vi "Autonomous Independent_04042012.vi"() -> ()   [LabVIEW 2011]
doc: "This VI is called when autonomous begins, and will automatically be terminated when autonomous ends. You can carry out timed or sensor driven robot movement independently without needing to return to the caller."
uses:
  <vilib>/Rock Robotics/WPI/Joystick/WPI_JoystickButtonState.ctl
  Robot Global Data.vi
  <vilib>/addons/control/pid/pid.llb/PID (DBL).vi
  <vilib>/Rock Robotics/WPI/RobotDrive/WPI_RobotDriveArcadeDrive_Standard(NoSaturation).vi
  <vilib>/addons/control/pid/NI_PID_pid.lvlib
panel:
  in  "Forward_Time_Cntrl_2_s2_p0":i32(slide) scale=0.0..100.0
  in  "Turn_Time_Cntrl_s2_p0":i32(slide) scale=0.0..100.0
  in  "Backward_Time_Cntrl_s2_p0":i32(slide) scale=0.0..100.0
  in  "Shooting_Time_Cntrl_s2_p0":u32(slide) scale=0.0..100.0
  in  "Shooting_Time_Cntrl_s1_p1":u32(slide) scale=0.0..100.0
  in  "Forward_Time_Cntrl_1_s1_p1":i32(slide) scale=0.0..100.0
  in  "Backward_Time_Cntrl_s1_p1":i32(slide) scale=0.0..100.0
  in  "Turn_Time_Cntrl_s1_p1":i32(slide) scale=0.0..100.0
  in  "Forward_Time_Cntrl_2_s1_p1":i32(slide) scale=0.0..100.0
  in  "Forward_Time_Cntrl_2_s1_p0":i32(slide)=15 scale=0.0..100.0
  in  "Turn_Time_Cntrl_s1_p0":i32(slide)=25 scale=0.0..100.0
  in  "Backward_Time_Cntrl_s1_p0":i32(slide)=81 scale=0.0..100.0
  in  "Forward_Time_Cntrl_1_s1_p0":i32(slide)=55 scale=0.0..100.0
  in  "Shooting_Time_Cntrl_s1_p0":u32(slide)=42 scale=0.0..100.0
  in  "Shooter_Speed_Cntrl":dbl(slide)=0.65 scale=-1.0..1.0
  in  "ARM_FWD_LIMIT":dbl(slide)=0.53 scale=1.0..-1.0
  in  "ARM_REV_LIMIT":dbl(slide)=-0.14110429447852763 scale=1.0..-1.0
  in  "ARM_HOME":dbl(slide)=0.53 scale=1.0..-1.0
  in  "Feeder_Arm_Speed":dbl
  out "JS1_BTNS":T1
  out "JS1_AXES":T2
  in  "Kinect_Arm_Conrol":dbl
  out "Kinect_Drive_Reduce":dbl=0.5
  out "KINECT_BTNS":T1
  out "LEFT_ARM_AXES":T2
  out "RIGHT_ARM_AXES":T2
  in  "Ball_Sucker_Speed":dbl(slide)=0.6 scale=-1.0..1.0
  in  "Feed_Speed_Cntrl":dbl(slide)=0.9 scale=-1.0..1.0
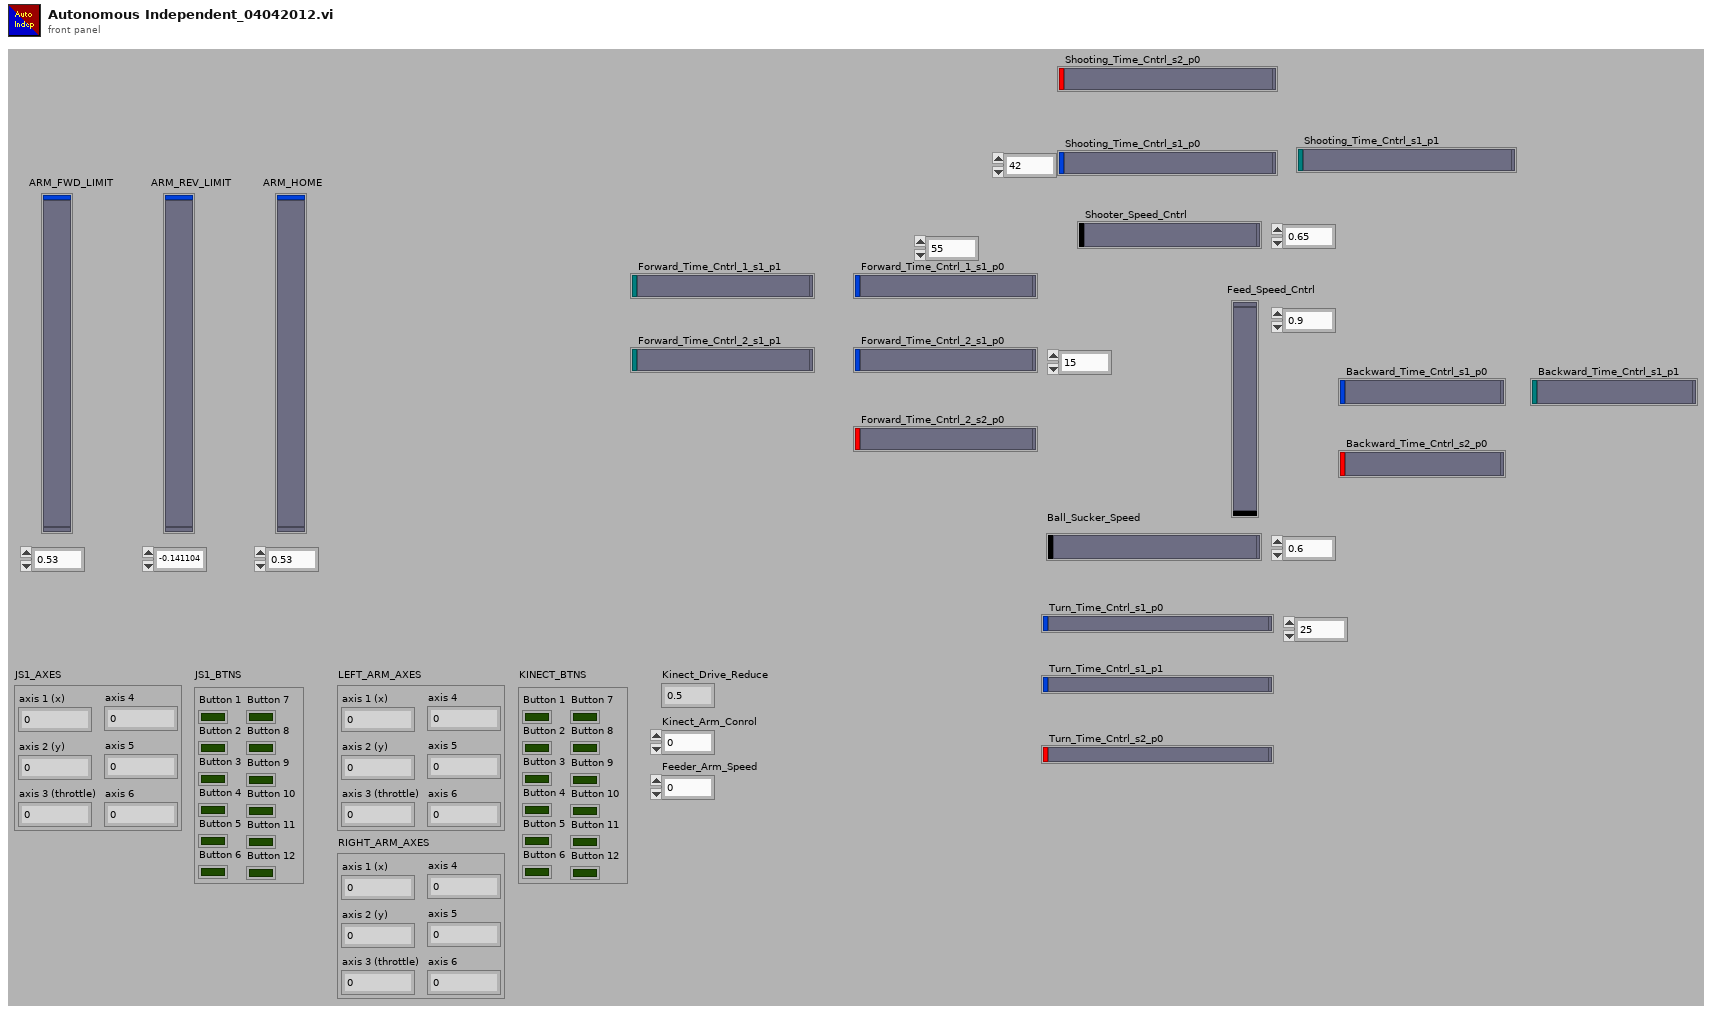
[diagram p1: front panel]
types:
  T1 = typedef "WPI_JoystickButtonState.ctl" = cluster{"Button 1":bool, "Button 2":bool, "Button 3":bool, "Button 4":bool, "Button 5":bool, "Button 6":bool, "Button 7":bool, "Button 8":bool, "Button 9":bool, "Button 10":bool, "Button 11":bool, "Button 12":bool}
  T2 = cluster{"axis 1 (x)":dbl, "axis 2 (y)":dbl, "axis 3 (throttle)":dbl, "axis 4":dbl, "axis 5":dbl, "axis 6":dbl}
  T3 = cluster{"proportional gain (Kc)":dbl, "integral time (Ti, min)":dbl, "derivative time (Td, min)":dbl}
  T4 = typedef "WPI_RobotDriveDevRef.ctl" = cluster{"DevStatus":errorcluster, "Motors[]":T5[], "Square Inputs":bool, "Max Output":dbl, "Isochronous":bool}
  T5 = typedef "WPI_MotorControlDeviceRef.ctl" = cluster{"DeviceStatus":errorcluster, "Type":enum16{"PWM", "CAN"}, "PWM":cluster{"Digital Module":T6, "PWM Channel":T7, "DeadBand":T8}, "CAN":cluster{"Device Number":u8, "Control Mode":T9, "Semaphore":T10, "Max Vout":dbl}, "Invert":bool, "TransformRef":T11, "InvTransformRef":T11}
  T6 = typedef "FPGA_TypedefDigitalModule.ctl" = enum16{"Digital Module 1", "Digital Module 2"}
  T7 = typedef "FPGA_DIOPWMChannel.ctl" = enum8{"PWM 1", "PWM 2", "PWM 3", "PWM 4", "PWM 5", "PWM 6", "PWM 7", "PWM 8", "PWM 9", "PWM 10", "Invalid"}
  T8 = typedef "WPI_PWMDeadband.ctl" = cluster{"Name":string, "maxPositivePwm":i32, "minPositivePwm":i32, "centerPwm":i32, "maxNegativePwm":i32, "minNegativePwm":i32, "angularRange":u16}
  T9 = typedef "WPI_CANJaguar_ControlMode.ctl" = enum8{"Percent VBus", "Current", "Speed", "Position", "Voltage"}
  T10 = typedef "Semaphore RefNum" = refnum<k1>
  T11 = typedef "WPI_PWMTransform_ConPane.ctl" = refnum<vi>
  T12 = typedef "WPI_JoystickDevRef.ctl" = cluster{"Device":T13}
  T13 = typedef "WPI_JoystickDeviceEnum.ctl" = enum16{"USB 1", "USB 2", "USB 3", "USB 4", "Kinect 1", "Kinect 2"}
  T14 = typedef "WPI_AnalogChannelDevRef.ctl" = cluster{"DevStatus":errorcluster, "Analog Module":T15, "Analog Channel":T16}
  T15 = typedef "FPGA_TypedefAnalogModule.ctl" = enum16{"Analog Module 1", "Analog Module 2"}
  T16 = typedef "FPGA_AIChannel.ctl" = enum8{"AI 1", "AI 2", "AI 3", "AI 4", "AI 5", "AI 6", "AI 7", "AI 8", "Invalid"}
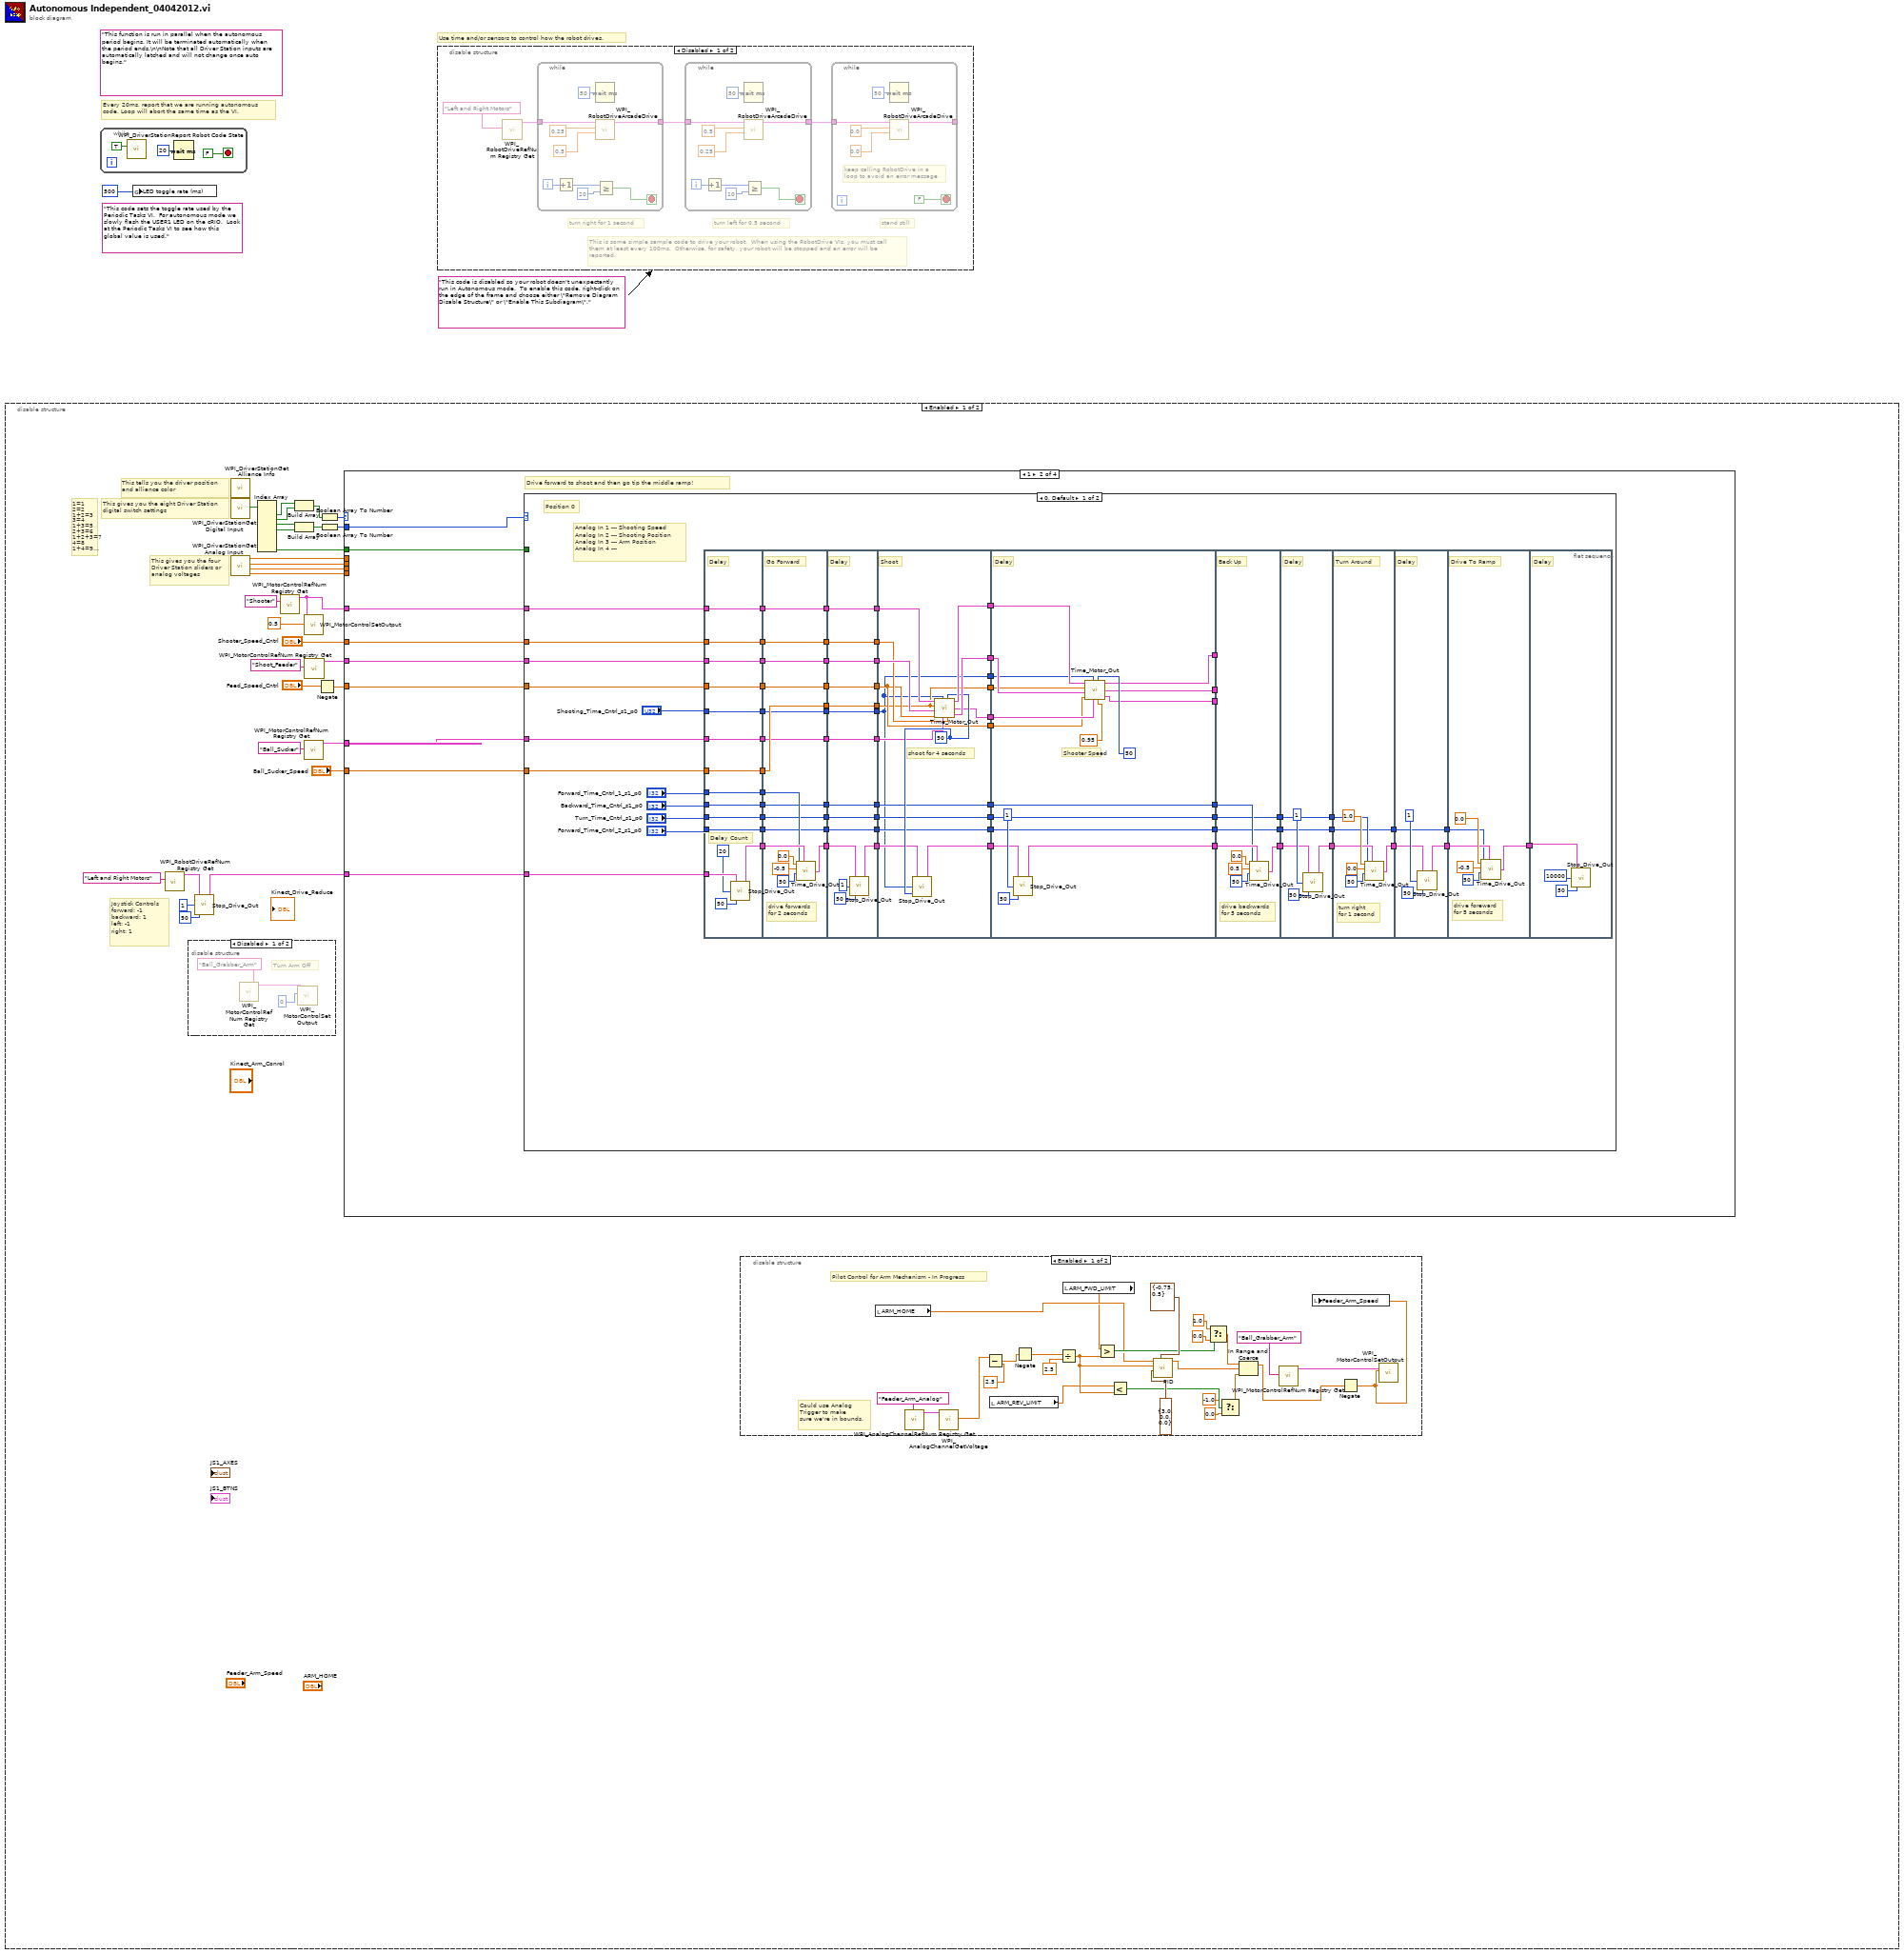
[diagram p0: block diagram]
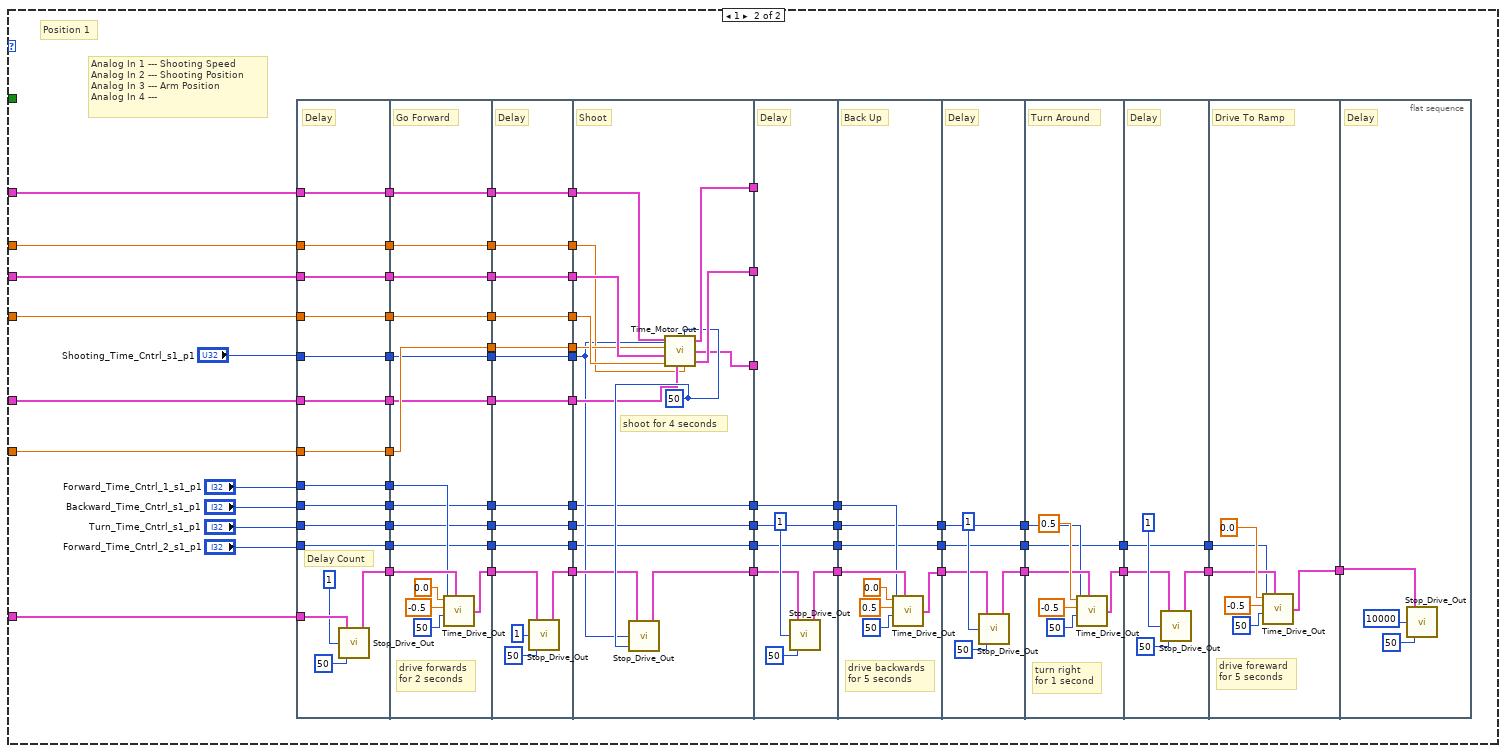
[diagram p5: hidden frame]
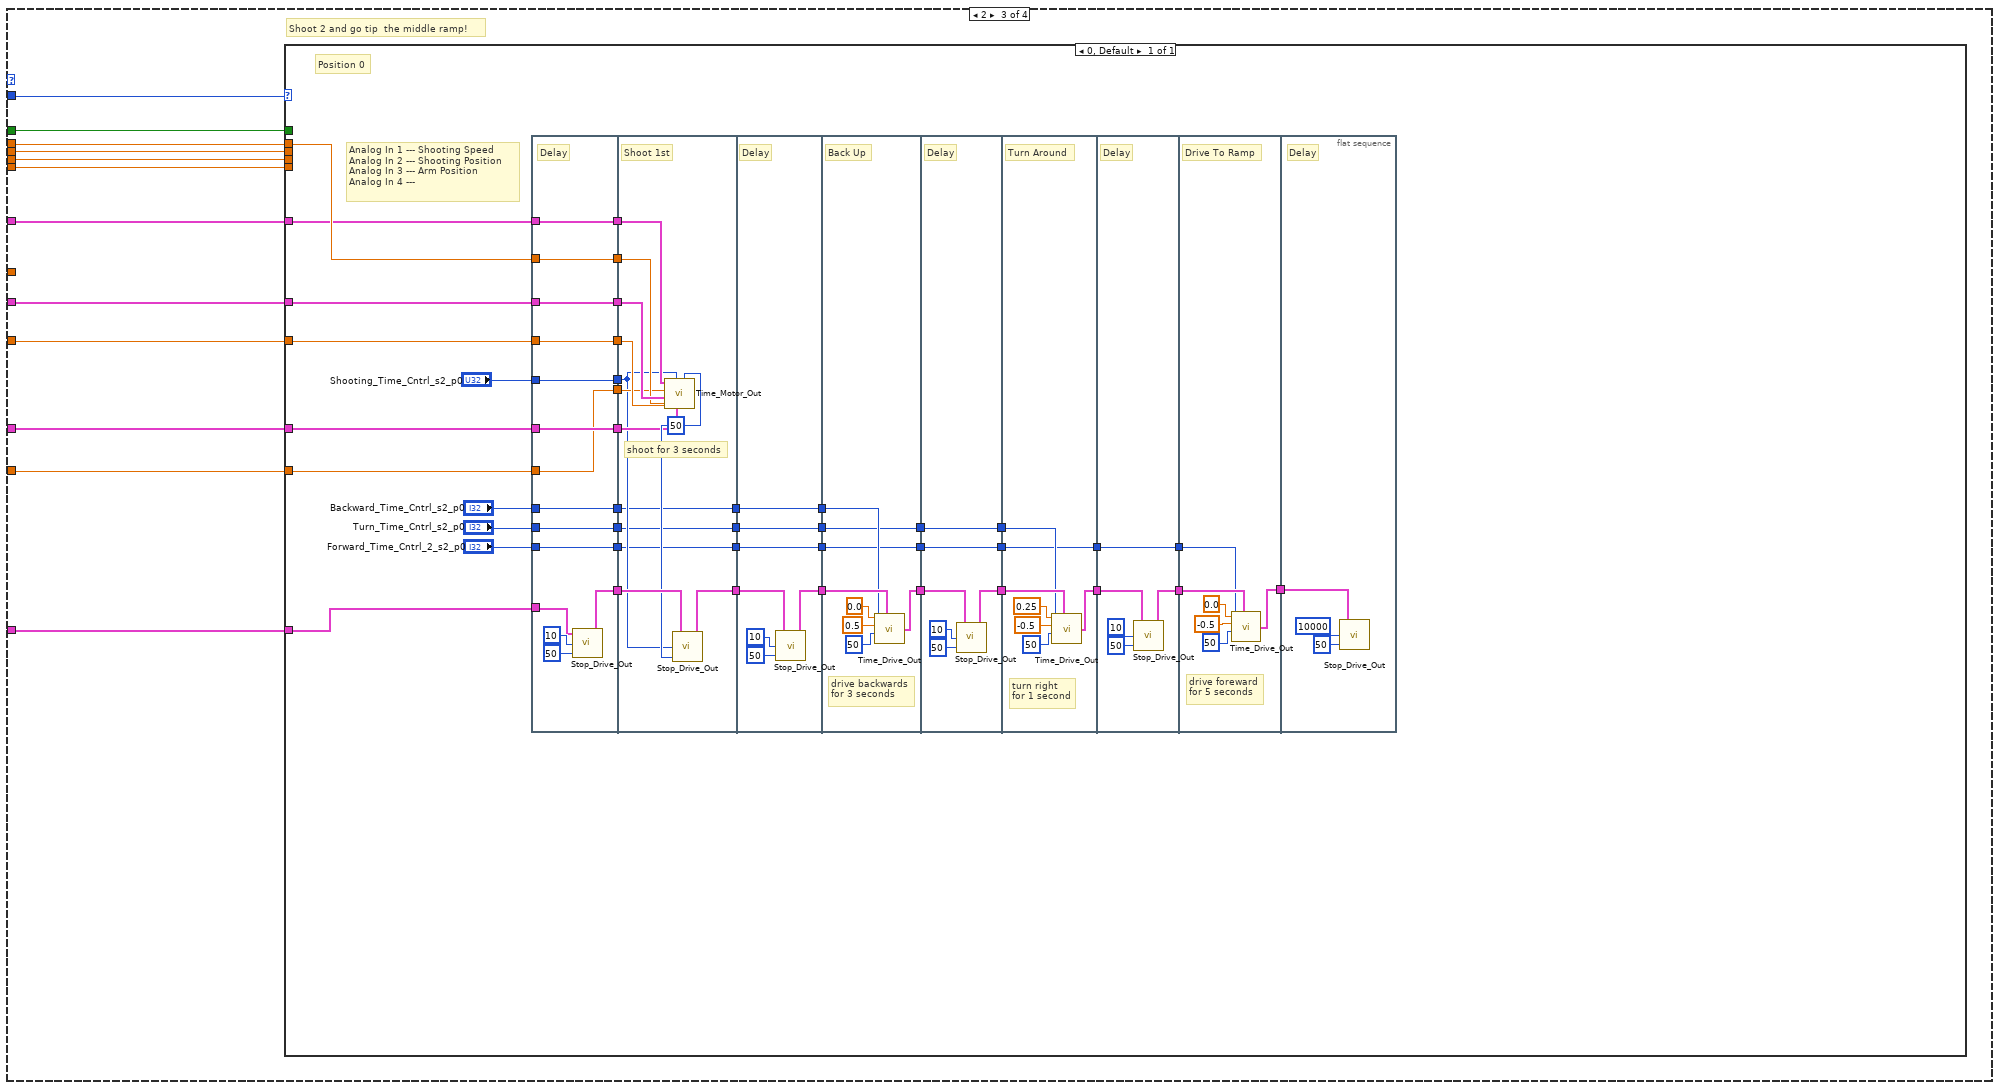
[diagram p6: hidden frame]
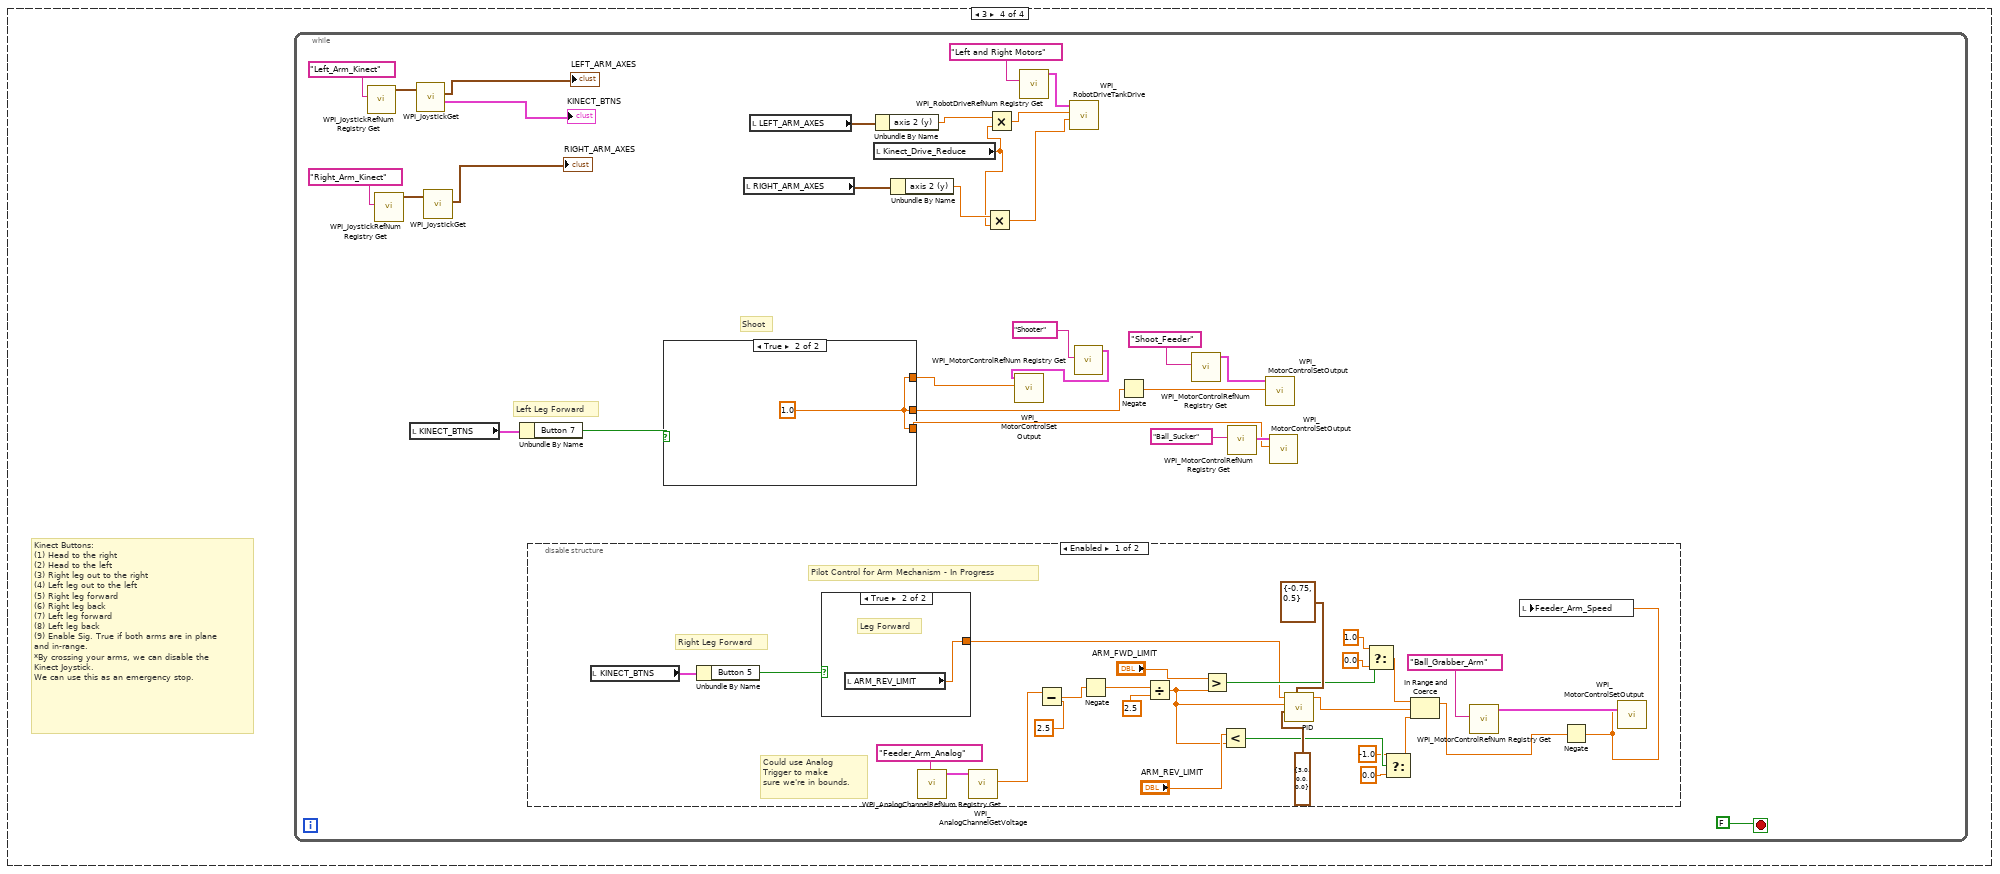
[diagram p7: hidden frame]
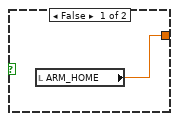
[diagram p8: hidden frame]
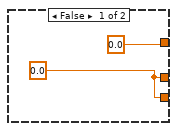
[diagram p10: hidden frame]
diagram:
  (unwired) "This code sets the toggle rate used by the Periodic Tasks VI.  For autonomous mode we slowly flash the USER1 LED on the cRIO.  Look at the Periodic Tasks VI to see how this global value is used."
  (unwired) "This code is disabled so your robot doesn't unexpectantly run in Autonomous mode.  To enable this code, right-click on the edge of the frame and choose either \"Remove Diagram Disable Structure\" or \"Enable This Subdiagram\"."
  (unwired) "This function is run in parallel when the autonomous period begins. It will be terminated automatically when the period ends.\n\nNote that all Driver Station inputs are automatically latched and will not change once auto begins."
  # "Every 20ms, report that we are running autonomous\ncode. Loop will abort the same time as the VI."
  # "Use time and/or sensors to control how the robot drives."
  n1 = disable-structure shown="Enabled" {
    frame Enabled {
      # "Joystick Controls\nforward: -1\nbackward: 1\nleft: -1\nright: 1"
      # "1=1\n2=2\n1+2=3\n3=4\n1+3=5\n2+3=6\n1+2+3=7\n4=8\n1+4=9\n2+4=10\n1+2+4=11\n3+4=12\n1+3+4=13\n2+3+4=14\n1+2+3+4=15"
      # "This tells you the driver position\nand alliance color"
      # "This gives you the eight Driver Station\ndigital switch settings"
      # "This gives you the four\nDriver Station sliders or\nanalog voltages"
      n2 = call <vilib>:"WPI_RobotDriveRefNum Registry Get.vi"("refnum name"="Left and Right Motors") -> ("RobotDriveDevRef"=w13:T4)  [unwired: 1 in, 9 out]
      n3 = disable-structure shown="Disabled" {
        frame Disabled {
          # "Turn Arm Off"
          n4 = call <vilib>:"WPI_MotorControlRefNum Registry Get.vi"("refnum name"="Ball_Grabber_Arm") -> ("MotorControlDevRef"=w60:T5)  [unwired: 1 in, 9 out]
          n5 = call <vilib>:"WPI_MotorControlSetOutput.vi"("Output"=0, "MotorControlDevRef"=w60) -> ()  [unwired: 3 in, 7 out]
        }
        frame Enabled {
        }
      }
      n6 = call "Stop_Drive_Out.vi"("Step_Duration_ms"=50, "Num_Steps"=u32 1 ("milliseconds to wait"), "Drive_In"=w13) -> ("Drive_Out"=w12:T4)
      n7 = call <vilib>:"WPI_DriverStationGet Alliance Info.vi"() -> ()  [unwired: 12 out]
      n8 = call <vilib>:"WPI_DriverStationGet Digital Input.vi"() -> ("Driver Station Digital Input (1-8)"=w31:bool[])  [unwired: 11 out]
      n9 = call <vilib>:"WPI_DriverStationGet Analog Input.vi"() -> ("Analog 4 (V)"=w28:dbl, "Analog 3 (V)"=w29:dbl, "Analog 2 (V)"=w16:dbl, "Analog 1 (V)"=w17:dbl)  [unwired: 8 out]
      n10 = Index Array(array=w31) -> (element #1=w20:bool, element #2=w19:bool, element #3=w22:bool, element #4=w21:bool, element #8=w27:bool)  [unwired: 8 in, 3 out]
      n11 = call <vilib>:"WPI_MotorControlRefNum Registry Get.vi"("refnum name"="Shooter") -> ("MotorControlDevRef"=w3:T5)  [unwired: 9 in, 1 out]
      n12 = Build Array(w20, w19) -> (w18:bool[])
      n13 = Build Array(w22, w21) -> (w30:bool[])
      n14 = call <vilib>:"WPI_MotorControlSetOutput.vi"("Output"=0.5, "MotorControlDevRef"=w3) -> ()  [unwired: 8 in, 2 out]
      n15 = call <vilib>:"WPI_MotorControlRefNum Registry Get.vi"("refnum name"="Ball_Sucker") -> ("MotorControlDevRef"=w6:T5)  [unwired: 9 in, 1 out]
      n16 = call <vilib>:"WPI_MotorControlRefNum Registry Get.vi"("refnum name"="Shoot_Feeder") -> ("MotorControlDevRef"=w24:T5)  [unwired: 9 in, 1 out]
      n17 = Negate(x="Feed_Speed_Cntrl") -> (-x=w8:dbl)
      n18 = Boolean Array To Number(Boolean array=w18) -> (number=w11:u32)
      n19 = Boolean Array To Number(Boolean array=w30) -> (number=w10:u32)
      n20 = case shown="1" w11 {
        tunnel: w17 -> [_ _ w439 _]
        tunnel: w16 -> [_ _ w438 _]
        tunnel: w29 -> [_ _ w437 _]
        tunnel: w28 -> [_ _ w436 _]
        tunnel: w27 -> [_ w69 w440 _]
        tunnel: w8 -> [_ w68 w435 _]
        tunnel: w3 -> [_ w67 w434 _]
        tunnel: w24 -> [_ w66 w433 _]
        tunnel: w12 -> [_ w65 w432 _]
        tunnel: w10 -> [_ w64 w431 _]
        tunnel: w6 -> [_ w63 w429 _]
        tunnel: "Ball_Sucker_Speed" -> [_ w62 w430 _]
        tunnel: "Shooter_Speed_Cntrl" -> [_ w61 _ _]
        frame 0, Default {
          # "Stop Motors"
        }
        frame 1 {
          # "Drive forward to shoot and then go tip the middle ramp!"
          n21 = case shown="0, Default" w64 {
            tunnel: w69 -> [_ _]
            tunnel: w68 -> [w143 w325]
            tunnel: w67 -> [w142 w324]
            tunnel: w66 -> [w141 w323]
            tunnel: w65 -> [w140 w322]
            tunnel: w63 -> [w139 w321]
            tunnel: w62 -> [w138 w320]
            tunnel: w61 -> [w106 w288]
            frame 0, Default {
              # "Analog In 1 --- Shooting Speed\nAnalog In 2 --- Shooting Position\nAnalog In 3 --- Arm Position\nAnalog In 4 ---"
              # "Position 0"
              n22 = flat-sequence {
                tunnel: [w153] -> w137
                tunnel: [w158] -> w136
                tunnel: [w157] -> w135
                tunnel: [w156] -> w134
                tunnel: [w155] -> w133
                tunnel: w142 -> [w156]
                tunnel: w141 -> [w157]
                tunnel: w106 -> [w155]
                tunnel: w143 -> [w158]
                tunnel: w140 -> [w152]
                tunnel: [w151] -> w132
                tunnel: w138 -> [w151]
                tunnel: [w150] -> w131
                tunnel: w139 -> [w150]
                tunnel: [w148] -> w103
                tunnel: "Shooting_Time_Cntrl_s1_p0" -> [w148]
                tunnel: "Forward_Time_Cntrl_1_s1_p0" -> [w147]
                tunnel: [w147] -> w102
                tunnel: "Backward_Time_Cntrl_s1_p0" -> [w146]
                tunnel: [w146] -> w101
                tunnel: "Turn_Time_Cntrl_s1_p0" -> [w145]
                tunnel: [w145] -> w90
                tunnel: [w144] -> w87
                tunnel: "Forward_Time_Cntrl_2_s1_p0" -> [w144]
                tunnel: w137 -> [w171]
                tunnel: [w170] -> w130
                tunnel: [w169] -> w129
                tunnel: w136 -> [w169]
                tunnel: [w168] -> w128
                tunnel: w135 -> [w168]
                tunnel: [w167] -> w127
                tunnel: w134 -> [w167]
                tunnel: [w166] -> w126
                tunnel: w133 -> [w166]
                tunnel: w132 -> [w165]
                tunnel: [w165] -> w125
                tunnel: w131 -> [w164]
                tunnel: [w164] -> w124
                tunnel: [w163] -> w104
                tunnel: w103 -> [w163]
                tunnel: w102 -> [w162]
                tunnel: w101 -> [w161]
                tunnel: [w161] -> w100
                tunnel: [w160] -> w91
                tunnel: w90 -> [w160]
                tunnel: [w159] -> w88
                tunnel: w87 -> [w159]
                tunnel: w130 -> [w182]
                tunnel: [w181] -> w123
                tunnel: [w188] -> w122
                tunnel: w129 -> [w188]
                tunnel: [w187] -> w121
                tunnel: w128 -> [w187]
                tunnel: [w186] -> w120
                tunnel: w127 -> [w186]
                tunnel: [w185] -> w119
                tunnel: w126 -> [w185]
                tunnel: [w180] -> w118
                tunnel: w125 -> [w180]
                tunnel: [w179] -> w117
                tunnel: w124 -> [w179]
                tunnel: [w178] -> w105
                tunnel: w104 -> [w178]
                tunnel: w100 -> [w177]
                tunnel: [w177] -> w99
                tunnel: [w176] -> w92
                tunnel: w91 -> [w176]
                tunnel: [w175] -> w89
                tunnel: w88 -> [w175]
                tunnel: w123 -> [w199]
                tunnel: [w198] -> w116
                tunnel: w122 -> [w191]
                tunnel: w121 -> [w204]
                tunnel: [w203] -> w115
                tunnel: [w202] -> w114
                tunnel: w120 -> [w201]
                tunnel: w119 -> [w195]
                tunnel: [w197] -> w113
                tunnel: w118 -> [w190]
                tunnel: w117 -> [w196]
                tunnel: w105 -> [w189]
                tunnel: w99 -> [w194]
                tunnel: [w194] -> w98
                tunnel: [w193] -> w93
                tunnel: w92 -> [w193]
                tunnel: w89 -> [w192]
                tunnel: [w192] -> w81
                tunnel: [w191] -> w72
                tunnel: [w190] -> w71
                tunnel: [w189] -> w70
                tunnel: w116 -> [w220]
                tunnel: [w219] -> w112
                tunnel: w115 -> [w213]
                tunnel: w114 -> [w214]
                tunnel: w113 -> [w212]
                tunnel: w98 -> [w218]
                tunnel: [w218] -> w97
                tunnel: [w217] -> w94
                tunnel: w93 -> [w217]
                tunnel: [w216] -> w82
                tunnel: w81 -> [w216]
                tunnel: [w211] -> w75
                tunnel: [w210] -> w74
                tunnel: [w209] -> w73
                tunnel: w72 -> [w208]
                tunnel: w71 -> [w207]
                tunnel: w70 -> [w206]
                tunnel: w112 -> [w227]
                tunnel: [w226] -> w111
                tunnel: w97 -> [w225]
                tunnel: [w224] -> w95
                tunnel: w94 -> [w224]
                tunnel: [w223] -> w83
                tunnel: w82 -> [w223]
                tunnel: w75 -> [_]
                tunnel: w74 -> [_]
                tunnel: w73 -> [_]
                tunnel: w111 -> [w234]
                tunnel: [w233] -> w110
                tunnel: [w232] -> w96
                tunnel: w95 -> [w232]
                tunnel: [w231] -> w84
                tunnel: w83 -> [w231]
                tunnel: [w239] -> w109
                tunnel: w110 -> [w240]
                tunnel: w96 -> [w238]
                tunnel: [w237] -> w85
                tunnel: w84 -> [w237]
                tunnel: w109 -> [w246]
                tunnel: [w245] -> w108
                tunnel: [w244] -> w86
                tunnel: w85 -> [w244]
                tunnel: w108 -> [w251]
                tunnel: [w250] -> w107
                tunnel: w86 -> [w249]
                tunnel: w107 -> [w255]
                frame #0 {
                  # "Delay Count"
                  # "Delay"
                  n23 = call "Stop_Drive_Out.vi"("Step_Duration_ms"=50, "Num_Steps"=u32 20 ("milliseconds to wait"), "Drive_In"=w152) -> ("Drive_Out"=w153:T4)
                }
                frame #1 {
                  # "drive forwards\nfor 2 seconds"
                  # "Go Forward"
                  n24 = call "Time_Drive_Out.vi"("X_Axis"=0.0 ("X axis value"), "Y_Axis"=-0.5 ("X axis value"), "Step_Duration_ms"=u32 50 ("milliseconds to wait"), "Num_Steps"=w162, "Drive_In"=w171) -> ("Drive_Out"=w170:T4)
                }
                frame #2 {
                  # "Delay"
                  n25 = call "Stop_Drive_Out.vi"("Step_Duration_ms"=50, "Num_Steps"=u32 1 ("milliseconds to wait"), "Drive_In"=w182) -> ("Drive_Out"=w181:T4)
                }
                frame #3 {
                  w200 = 50
                  # "Shoot"
                  # "shoot for 4 seconds"
                  n26 = call "Stop_Drive_Out.vi"("Step_Duration_ms"=w200, "Num_Steps"=w189, "Drive_In"=w199) -> ("Drive_Out"=w198:T4)
                  n27 = call "Time_Motor_Out.vi"("Motor_1_Speed"=w195, "Step_Duration_ms"=w200, "Motor_3"=w196, "Motor_2_Speed"=w191, "Motor_2"=w204, "Num_Steps"=w189, "Motor_3_Speed"=w190, "Motor_1"=w201) -> ("Motor_2_Out"=w203:T5, "Motor_3_Out"=w197:T5, "Motor_1_Out"=w202:T5)
                }
                frame #4 {
                  # "Shooter Speed"
                  # "Delay"
                  n28 = call "Stop_Drive_Out.vi"("Step_Duration_ms"=50, "Num_Steps"=u32 1 ("milliseconds to wait"), "Drive_In"=w220) -> ("Drive_Out"=w219:T4)
                  n29 = call "Time_Motor_Out.vi"("Motor_1_Speed"=0.95, "Step_Duration_ms"=50, "Motor_3"=w212, "Motor_2_Speed"=w208, "Motor_2"=w213, "Num_Steps"=w206, "Motor_3_Speed"=w207, "Motor_1"=w214) -> ("Motor_2_Out"=w209:T5, "Motor_3_Out"=w210:T5, "Motor_1_Out"=w211:T5)
                }
                frame #5 {
                  # "Back Up"
                  # "drive backwards\nfor 5 seconds"
                  n30 = call "Time_Drive_Out.vi"("X_Axis"=0.0 ("X axis value"), "Y_Axis"=0.5 ("X axis value"), "Step_Duration_ms"=u32 50 ("milliseconds to wait"), "Num_Steps"=w225, "Drive_In"=w227) -> ("Drive_Out"=w226:T4)
                }
                frame #6 {
                  # "Delay"
                  n31 = call "Stop_Drive_Out.vi"("Step_Duration_ms"=50, "Num_Steps"=u32 1 ("milliseconds to wait"), "Drive_In"=w234) -> ("Drive_Out"=w233:T4)
                }
                frame #7 {
                  # "turn right\nfor 1 second"
                  # "Turn Around"
                  n32 = call "Time_Drive_Out.vi"("X_Axis"=1.0 ("X axis value"), "Y_Axis"=0.0 ("X axis value"), "Step_Duration_ms"=u32 50 ("milliseconds to wait"), "Num_Steps"=w238, "Drive_In"=w240) -> ("Drive_Out"=w239:T4)
                }
                frame #8 {
                  # "Delay"
                  n33 = call "Stop_Drive_Out.vi"("Step_Duration_ms"=50, "Num_Steps"=u32 1 ("milliseconds to wait"), "Drive_In"=w246) -> ("Drive_Out"=w245:T4)
                }
                frame #9 {
                  # "drive foreward\nfor 5 seconds"
                  # "Drive To Ramp"
                  n34 = call "Time_Drive_Out.vi"("X_Axis"=0.0 ("X axis value"), "Y_Axis"=-0.5 ("X axis value"), "Step_Duration_ms"=u32 50 ("milliseconds to wait"), "Num_Steps"=w249, "Drive_In"=w251) -> ("Drive_Out"=w250:T4)
                }
                frame #10 {
                  # "Delay"
                  n35 = call "Stop_Drive_Out.vi"("Step_Duration_ms"=50, "Num_Steps"=u32 10000 ("milliseconds to wait"), "Drive_In"=w255) -> ()  [unwired: 1 out]
                }
              }
            }
            frame 1 {
              # "Analog In 1 --- Shooting Speed\nAnalog In 2 --- Shooting Position\nAnalog In 3 --- Arm Position\nAnalog In 4 ---"
              # "Position 1"
              n36 = flat-sequence {
                tunnel: [w335] -> w319
                tunnel: [w340] -> w318
                tunnel: [w339] -> w317
                tunnel: [w338] -> w316
                tunnel: [w337] -> w315
                tunnel: w324 -> [w338]
                tunnel: w323 -> [w339]
                tunnel: w288 -> [w337]
                tunnel: w325 -> [w340]
                tunnel: w322 -> [w334]
                tunnel: [w333] -> w314
                tunnel: w320 -> [w333]
                tunnel: [w332] -> w313
                tunnel: w321 -> [w332]
                tunnel: [w330] -> w285
                tunnel: "Shooting_Time_Cntrl_s1_p1" -> [w330]
                tunnel: "Forward_Time_Cntrl_1_s1_p1" -> [w329]
                tunnel: [w329] -> w284
                tunnel: "Backward_Time_Cntrl_s1_p1" -> [w328]
                tunnel: [w328] -> w283
                tunnel: "Turn_Time_Cntrl_s1_p1" -> [w327]
                tunnel: [w327] -> w272
                tunnel: [w326] -> w269
                tunnel: "Forward_Time_Cntrl_2_s1_p1" -> [w326]
                tunnel: w319 -> [w353]
                tunnel: [w352] -> w312
                tunnel: [w351] -> w311
                tunnel: w318 -> [w351]
                tunnel: [w350] -> w310
                tunnel: w317 -> [w350]
                tunnel: [w349] -> w309
                tunnel: w316 -> [w349]
                tunnel: [w348] -> w308
                tunnel: w315 -> [w348]
                tunnel: w314 -> [w347]
                tunnel: [w347] -> w307
                tunnel: w313 -> [w346]
                tunnel: [w346] -> w306
                tunnel: [w345] -> w286
                tunnel: w285 -> [w345]
                tunnel: w284 -> [w344]
                tunnel: w283 -> [w343]
                tunnel: [w343] -> w282
                tunnel: [w342] -> w273
                tunnel: w272 -> [w342]
                tunnel: [w341] -> w270
                tunnel: w269 -> [w341]
                tunnel: w312 -> [w364]
                tunnel: [w363] -> w305
                tunnel: [w370] -> w304
                tunnel: w311 -> [w370]
                tunnel: [w369] -> w303
                tunnel: w310 -> [w369]
                tunnel: [w368] -> w302
                tunnel: w309 -> [w368]
                tunnel: [w367] -> w301
                tunnel: w308 -> [w367]
                tunnel: [w362] -> w300
                tunnel: w307 -> [w362]
                tunnel: [w361] -> w299
                tunnel: w306 -> [w361]
                tunnel: [w360] -> w287
                tunnel: w286 -> [w360]
                tunnel: w282 -> [w359]
                tunnel: [w359] -> w281
                tunnel: [w358] -> w274
                tunnel: w273 -> [w358]
                tunnel: [w357] -> w271
                tunnel: w270 -> [w357]
                tunnel: w305 -> [w380]
                tunnel: [w379] -> w298
                tunnel: w304 -> [w386]
                tunnel: w303 -> [w385]
                tunnel: [w384] -> w297
                tunnel: [w383] -> w296
                tunnel: w302 -> [w382]
                tunnel: w301 -> [w375]
                tunnel: [w378] -> w295
                tunnel: w300 -> [w377]
                tunnel: w299 -> [w376]
                tunnel: w287 -> [w374]
                tunnel: w281 -> [w373]
                tunnel: [w373] -> w280
                tunnel: [w372] -> w275
                tunnel: w274 -> [w372]
                tunnel: w271 -> [w371]
                tunnel: [w371] -> w263
                tunnel: w298 -> [w391]
                tunnel: [w390] -> w294
                tunnel: w297 -> [_]
                tunnel: w296 -> [_]
                tunnel: w295 -> [_]
                tunnel: w280 -> [w389]
                tunnel: [w389] -> w279
                tunnel: [w388] -> w276
                tunnel: w275 -> [w388]
                tunnel: [w387] -> w264
                tunnel: w263 -> [w387]
                tunnel: w294 -> [w398]
                tunnel: [w397] -> w293
                tunnel: w279 -> [w396]
                tunnel: [w395] -> w277
                tunnel: w276 -> [w395]
                tunnel: [w394] -> w265
                tunnel: w264 -> [w394]
                tunnel: w293 -> [w405]
                tunnel: [w404] -> w292
                tunnel: [w403] -> w278
                tunnel: w277 -> [w403]
                tunnel: [w402] -> w266
                tunnel: w265 -> [w402]
                tunnel: [w410] -> w291
                tunnel: w292 -> [w411]
                tunnel: w278 -> [w409]
                tunnel: [w408] -> w267
                tunnel: w266 -> [w408]
                tunnel: w291 -> [w417]
                tunnel: [w416] -> w290
                tunnel: [w415] -> w268
                tunnel: w267 -> [w415]
                tunnel: w290 -> [w422]
                tunnel: [w421] -> w289
                tunnel: w268 -> [w420]
                tunnel: w289 -> [w426]
                frame #0 {
                  # "Delay Count"
                  # "Delay"
                  n37 = call "Stop_Drive_Out.vi"("Step_Duration_ms"=50, "Num_Steps"=u32 1 ("milliseconds to wait"), "Drive_In"=w334) -> ("Drive_Out"=w335:T4)
                }
                frame #1 {
                  # "drive forwards\nfor 2 seconds"
                  # "Go Forward"
                  n38 = call "Time_Drive_Out.vi"("X_Axis"=0.0 ("X axis value"), "Y_Axis"=-0.5 ("X axis value"), "Step_Duration_ms"=u32 50 ("milliseconds to wait"), "Num_Steps"=w344, "Drive_In"=w353) -> ("Drive_Out"=w352:T4)
                }
                frame #2 {
                  # "Delay"
                  n39 = call "Stop_Drive_Out.vi"("Step_Duration_ms"=50, "Num_Steps"=u32 1 ("milliseconds to wait"), "Drive_In"=w364) -> ("Drive_Out"=w363:T4)
                }
                frame #3 {
                  w381 = 50
                  # "Shoot"
                  # "shoot for 4 seconds"
                  n40 = call "Stop_Drive_Out.vi"("Step_Duration_ms"=w381, "Num_Steps"=w374, "Drive_In"=w380) -> ("Drive_Out"=w379:T4)
                  n41 = call "Time_Motor_Out.vi"("Motor_1_Speed"=w375, "Step_Duration_ms"=w381, "Motor_3"=w376, "Motor_2_Speed"=w386, "Motor_2"=w385, "Num_Steps"=w374, "Motor_3_Speed"=w377, "Motor_1"=w382) -> ("Motor_2_Out"=w384:T5, "Motor_3_Out"=w378:T5, "Motor_1_Out"=w383:T5)
                }
                frame #4 {
                  # "Delay"
                  n42 = call "Stop_Drive_Out.vi"("Step_Duration_ms"=50, "Num_Steps"=u32 1 ("milliseconds to wait"), "Drive_In"=w391) -> ("Drive_Out"=w390:T4)
                }
                frame #5 {
                  # "Back Up"
                  # "drive backwards\nfor 5 seconds"
                  n43 = call "Time_Drive_Out.vi"("X_Axis"=0.0 ("X axis value"), "Y_Axis"=0.5 ("X axis value"), "Step_Duration_ms"=u32 50 ("milliseconds to wait"), "Num_Steps"=w396, "Drive_In"=w398) -> ("Drive_Out"=w397:T4)
                }
                frame #6 {
                  # "Delay"
                  n44 = call "Stop_Drive_Out.vi"("Step_Duration_ms"=50, "Num_Steps"=u32 1 ("milliseconds to wait"), "Drive_In"=w405) -> ("Drive_Out"=w404:T4)
                }
                frame #7 {
                  # "turn right\nfor 1 second"
                  # "Turn Around"
                  n45 = call "Time_Drive_Out.vi"("X_Axis"=0.5 ("X axis value"), "Y_Axis"=-0.5 ("X axis value"), "Step_Duration_ms"=u32 50 ("milliseconds to wait"), "Num_Steps"=w409, "Drive_In"=w411) -> ("Drive_Out"=w410:T4)
                }
                frame #8 {
                  # "Delay"
                  n46 = call "Stop_Drive_Out.vi"("Step_Duration_ms"=50, "Num_Steps"=u32 1 ("milliseconds to wait"), "Drive_In"=w417) -> ("Drive_Out"=w416:T4)
                }
                frame #9 {
                  # "drive foreward\nfor 5 seconds"
                  # "Drive To Ramp"
                  n47 = call "Time_Drive_Out.vi"("X_Axis"=0.0 ("X axis value"), "Y_Axis"=-0.5 ("X axis value"), "Step_Duration_ms"=u32 50 ("milliseconds to wait"), "Num_Steps"=w420, "Drive_In"=w422) -> ("Drive_Out"=w421:T4)
                }
                frame #10 {
                  # "Delay"
                  n48 = call "Stop_Drive_Out.vi"("Step_Duration_ms"=50, "Num_Steps"=u32 10000 ("milliseconds to wait"), "Drive_In"=w426) -> ()  [unwired: 1 out]
                }
              }
            }
          }
        }
        frame 2 {
          # "Shoot 2 and go tip  the middle ramp!"
          n49 = case shown="0, Default" w431 {
            tunnel: w440 -> [_]
            tunnel: w439 -> [w481]
            tunnel: w438 -> [_]
            tunnel: w437 -> [_]
            tunnel: w436 -> [_]
            tunnel: w435 -> [w480]
            tunnel: w434 -> [w479]
            tunnel: w433 -> [w478]
            tunnel: w432 -> [w477]
            tunnel: w429 -> [w461]
            tunnel: w430 -> [w476]
            frame 0, Default {
              # "Analog In 1 --- Shooting Speed\nAnalog In 2 --- Shooting Position\nAnalog In 3 --- Arm Position\nAnalog In 4 ---"
              # "Position 0"
              n50 = flat-sequence {
                tunnel: [w495] -> w475
                tunnel: [w494] -> w474
                tunnel: [w491] -> w473
                tunnel: [w493] -> w472
                tunnel: [w492] -> w471
                tunnel: w479 -> [w495]
                tunnel: w478 -> [w494]
                tunnel: w481 -> [w493]
                tunnel: w480 -> [w492]
                tunnel: w477 -> [w488]
                tunnel: w461 -> [w487]
                tunnel: [w487] -> w470
                tunnel: [w486] -> w469
                tunnel: w476 -> [w486]
                tunnel: [w485] -> w460
                tunnel: "Shooting_Time_Cntrl_s2_p0" -> [w485]
                tunnel: [w484] -> w456
                tunnel: "Backward_Time_Cntrl_s2_p0" -> [w484]
                tunnel: [w483] -> w450
                tunnel: "Turn_Time_Cntrl_s2_p0" -> [w483]
                tunnel: [w482] -> w442
                tunnel: "Forward_Time_Cntrl_2_s2_p0" -> [w482]
                tunnel: w475 -> [w508]
                tunnel: w474 -> [w507]
                tunnel: w473 -> [w504]
                tunnel: w472 -> [w505]
                tunnel: w471 -> [w506]
                tunnel: [w502] -> w468
                tunnel: w470 -> [w501]
                tunnel: w469 -> [w500]
                tunnel: w460 -> [w499]
                tunnel: [w498] -> w457
                tunnel: w456 -> [w498]
                tunnel: [w497] -> w451
                tunnel: w450 -> [w497]
                tunnel: [w496] -> w443
                tunnel: w442 -> [w496]
                tunnel: [w513] -> w467
                tunnel: w468 -> [w512]
                tunnel: [w511] -> w458
                tunnel: w457 -> [w511]
                tunnel: [w510] -> w452
                tunnel: w451 -> [w510]
                tunnel: [w509] -> w444
                tunnel: w443 -> [w509]
                tunnel: w467 -> [w520]
                tunnel: [w519] -> w466
                tunnel: w458 -> [w518]
                tunnel: [w517] -> w453
                tunnel: w452 -> [w517]
                tunnel: [w516] -> w445
                tunnel: w444 -> [w516]
                tunnel: w466 -> [w527]
                tunnel: [w526] -> w465
                tunnel: [w525] -> w454
                tunnel: w453 -> [w525]
                tunnel: [w524] -> w446
                tunnel: w445 -> [w524]
                tunnel: [w532] -> w464
                tunnel: w465 -> [w533]
                tunnel: w454 -> [w531]
                tunnel: [w530] -> w447
                tunnel: w446 -> [w530]
                tunnel: w464 -> [w539]
                tunnel: [w538] -> w463
                tunnel: [w537] -> w448
                tunnel: w447 -> [w537]
                tunnel: [w543] -> w462
                tunnel: w463 -> [w544]
                tunnel: w448 -> [w542]
                tunnel: w462 -> [w548]
                frame #0 {
                  # "Delay"
                  n51 = call "Stop_Drive_Out.vi"("Step_Duration_ms"=u32 50 ("milliseconds to wait"), "Num_Steps"=u32 10 ("milliseconds to wait"), "Drive_In"=w488) -> ("Drive_Out"=w491:T4)
                }
                frame #1 {
                  w503 = 50
                  # "shoot for 3 seconds"
                  # "Shoot 1st"
                  n52 = call "Time_Motor_Out.vi"("Motor_1_Speed"=w505, "Step_Duration_ms"=w503, "Motor_3"=w501, "Motor_2_Speed"=w506, "Motor_2"=w507, "Num_Steps"=w499, "Motor_3_Speed"=w500, "Motor_1"=w508) -> ()  [unwired: 3 out]
                  n53 = call "Stop_Drive_Out.vi"("Step_Duration_ms"=w503, "Num_Steps"=w499, "Drive_In"=w504) -> ("Drive_Out"=w502:T4)
                }
                frame #2 {
                  # "Delay"
                  n54 = call "Stop_Drive_Out.vi"("Step_Duration_ms"=u32 50 ("milliseconds to wait"), "Num_Steps"=u32 10 ("milliseconds to wait"), "Drive_In"=w512) -> ("Drive_Out"=w513:T4)
                }
                frame #3 {
                  # "drive backwards\nfor 3 seconds"
                  # "Back Up"
                  n55 = call "Time_Drive_Out.vi"("X_Axis"=0.0 ("X axis value"), "Y_Axis"=0.5 ("X axis value"), "Step_Duration_ms"=u32 50 ("milliseconds to wait"), "Num_Steps"=w518, "Drive_In"=w520) -> ("Drive_Out"=w519:T4)
                }
                frame #4 {
                  # "Delay"
                  n56 = call "Stop_Drive_Out.vi"("Step_Duration_ms"=u32 50 ("milliseconds to wait"), "Num_Steps"=u32 10 ("milliseconds to wait"), "Drive_In"=w527) -> ("Drive_Out"=w526:T4)
                }
                frame #5 {
                  # "turn right\nfor 1 second"
                  # "Turn Around"
                  n57 = call "Time_Drive_Out.vi"("X_Axis"=0.25 ("X axis value"), "Y_Axis"=-0.5 ("X axis value"), "Step_Duration_ms"=u32 50 ("milliseconds to wait"), "Num_Steps"=w531, "Drive_In"=w533) -> ("Drive_Out"=w532:T4)
                }
                frame #6 {
                  # "Delay"
                  n58 = call "Stop_Drive_Out.vi"("Step_Duration_ms"=u32 50 ("milliseconds to wait"), "Num_Steps"=u32 10 ("milliseconds to wait"), "Drive_In"=w539) -> ("Drive_Out"=w538:T4)
                }
                frame #7 {
                  # "drive foreward\nfor 5 seconds"
                  # "Drive To Ramp"
                  n59 = call "Time_Drive_Out.vi"("X_Axis"=0.0 ("X axis value"), "Y_Axis"=-0.5 ("X axis value"), "Step_Duration_ms"=u32 50 ("milliseconds to wait"), "Num_Steps"=w542, "Drive_In"=w544) -> ("Drive_Out"=w543:T4)
                }
                frame #8 {
                  # "Delay"
                  n60 = call "Stop_Drive_Out.vi"("Step_Duration_ms"=u32 50 ("milliseconds to wait"), "Num_Steps"=u32 10000 ("milliseconds to wait"), "Drive_In"=w548) -> ()  [unwired: 1 out]
                }
              }
            }
          }
        }
        frame 3 {
          # "Kinect Buttons:\n(1) Head to the right\n(2) Head to the left\n(3) Right leg out to the right\n(4) Left leg out to the left\n(5) Right leg forward\n(6) Right leg back\n(7) Left leg forward\n(8) Left leg back\n(9) Enable Sig. True if both arms are in plane and in-range.\n*By crossing your arms, we can disable the Kinect Joystick. \nWe can use this as an emergency stop."
          n61 = while {
            stop <- FALSE stop-if-true
            # "Left Leg Forward"
            # "Shoot"
            n62 = call <vilib>:"WPI_JoystickRefNum Registry Get.vi"("refnum name"="Left_Arm_Kinect") -> ("JoystickDevRef"=w576:T12)  [unwired: 1 in, 9 out]
            n63 = call <vilib>:"WPI_JoystickRefNum Registry Get.vi"("refnum name"="Right_Arm_Kinect") -> ("JoystickDevRef"=w574:T12)  [unwired: 1 in, 9 out]
            n64 = local read "KINECT_BTNS"() -> (w564:T1)
            n65 = call <vilib>:"WPI_JoystickGet.vi"("JoystickDevRef"=w576) -> ("Buttons"=→"KINECT_BTNS":T1, "Axes"=→"LEFT_ARM_AXES":T2)  [unwired: 1 in, 4 out]
            n66 = call <vilib>:"WPI_JoystickGet.vi"("JoystickDevRef"=w574) -> ("Axes"=→"RIGHT_ARM_AXES":T2)  [unwired: 1 in, 5 out]
            n67 = Unbundle By Name(w564) -> ("Button 7"=w563:bool)
            n68 = disable-structure shown="Enabled" {
              frame Enabled {
                # "Right Leg Forward"
                # "Could use Analog\nTrigger to make \nsure we're in bounds."
                # "Pilot Control for Arm Mechanism - In Progress"
                n69 = local read "KINECT_BTNS"() -> (w582:T1)
                n70 = Unbundle By Name(w582) -> ("Button 5"=w580:bool)
                n71 = case shown="True" w580 {
                  tunnel: [w608 w609] -> w581
                  frame False {
                    n72 = local read "ARM_HOME"() -> (w608:dbl)
                  }
                  frame True {
                    # "Leg Forward"
                    n73 = local read "ARM_REV_LIMIT"() -> (w609:dbl)
                  }
                }
                n74 = call <vilib>:"WPI_AnalogChannelRefNum Registry Get.vi"("refnum name"="Feeder_Arm_Analog") -> ("AIDeviceRef"=w606:T14)  [unwired: 1 in, 9 out]
                n75 = call <vilib>:"WPI_AnalogChannelGetVoltage.vi"("AIDeviceRef"=w606) -> ("Voltage"=w603:dbl)  [unwired: 1 in, 9 out]
                n76 = Subtract(x=w603, y=2.5) -> (x-y=w586:dbl)
                n77 = Negate(x=w586) -> (-x=w587:dbl)
                n78 = Divide(x=w587, y=2.5) -> (x/y=w584:dbl)
                n79 = Greater?(x="ARM_FWD_LIMIT", y=w584) -> (0:w598:bool)
                n80 = Less?(x="ARM_REV_LIMIT", y=w584) -> (x < y?=w600:bool)
                n81 = call-poly <vilib>:"PID.vi"("output range"=cluster{"output low":dbl, "output high":dbl} {"output low"=-0.75, "output high"=0.5}, "PID gains"=T3 {"proportional gain (Kc)"=3.0, "integral time (Ti, min)"=0.0, "derivative time (Td, min)"=0.0}, "process variable"=w584, "setpoint"=w581) -> ("output"=w591:dbl)  [unwired: 2 in, 5 out]
                n82 = Select(t=1.0, s=w598, f=0.0) -> (s? t:f=w596:dbl)
                n83 = Select(t=-1.0, s=w600, f=0.0) -> (s? t:f=w597:dbl)
                n84 = In Range and Coerce(upper limit=w596, x=w591, lower limit=w597) -> (coerced(x)=w583:dbl)  [unwired: 1 out]
                n85 = call <vilib>:"WPI_MotorControlRefNum Registry Get.vi"("refnum name"="Ball_Grabber_Arm") -> ("MotorControlDevRef"=w607:T5)  [unwired: 1 in, 9 out]
                n86 = Negate(x=w583) -> (-x=w588:dbl)
                n87 = local write "Feeder_Arm_Speed"(w588) -> ()
                n88 = call <vilib>:"WPI_MotorControlSetOutput.vi"("Output"=w588, "MotorControlDevRef"=w607) -> ()  [unwired: 3 in, 7 out]
              }
              frame Disabled {
              }
            }
            n89 = case shown="True" w563 {
              tunnel: [0.0 w612] -> w555
              tunnel: [w611 w612] -> w554
              tunnel: [w611 w612] -> w553
              frame False {
                w611 = 0.0
              }
              frame True {
                w612 = 1.0
              }
            }
            n90 = local read "RIGHT_ARM_AXES"() -> (w567:T2)
            n91 = local read "LEFT_ARM_AXES"() -> (w570:T2)
            n92 = local read "Kinect_Drive_Reduce"() -> (w565:dbl)
            n93 = Unbundle By Name(w570) -> ("axis 2 (y)"=w569:dbl)
            n94 = Unbundle By Name(w567) -> ("axis 2 (y)"=w566:dbl)
            n95 = Multiply(x=w566, y=w565) -> (x*y=w551:dbl)
            n96 = Multiply(x=w569, y=w565) -> (x*y=w568:dbl)
            n97 = call <vilib>:"WPI_RobotDriveRefNum Registry Get.vi"("refnum name"="Left and Right Motors") -> ("RobotDriveDevRef"=w571:T4)  [unwired: 1 in, 9 out]
            n98 = call <vilib>:"WPI_RobotDriveTankDrive.vi"("Right axis value"=w551, "Left axis value"=w568, "RobotDriveDevRef"=w571) -> ()  [unwired: 7 in, 2 out]
            n99 = call <vilib>:"WPI_MotorControlRefNum Registry Get.vi"("refnum name"="Shooter") -> ("MotorControlDevRef"=w561:T5)  [unwired: 9 in, 1 out]
            n100 = call <vilib>:"WPI_MotorControlSetOutput.vi"("Output"=w555, "MotorControlDevRef"=w561) -> ()  [unwired: 8 in, 2 out]
            n101 = Negate(x=w554) -> (-x=w558:dbl)
            n102 = call <vilib>:"WPI_MotorControlRefNum Registry Get.vi"("refnum name"="Shoot_Feeder") -> ("MotorControlDevRef"=w559:T5)  [unwired: 9 in, 1 out]
            n103 = call <vilib>:"WPI_MotorControlRefNum Registry Get.vi"("refnum name"="Ball_Sucker") -> ("MotorControlDevRef"=w556:T5)  [unwired: 9 in, 1 out]
            n104 = call <vilib>:"WPI_MotorControlSetOutput.vi"("Output"=w558, "MotorControlDevRef"=w559) -> ()  [unwired: 8 in, 2 out]
            n105 = call <vilib>:"WPI_MotorControlSetOutput.vi"("Output"=w553, "MotorControlDevRef"=w556) -> ()  [unwired: 8 in, 2 out]
          }
        }
      }
      n106 = disable-structure shown="Enabled" {
        frame Enabled {
          # "Could use Analog\nTrigger to make \nsure we're in bounds."
          # "Pilot Control for Arm Mechanism - In Progress"
          n107 = local read "ARM_HOME"() -> (w34:dbl)
          n108 = call <vilib>:"WPI_AnalogChannelRefNum Registry Get.vi"("refnum name"="Feeder_Arm_Analog") -> ("AIDeviceRef"=w56:T14)  [unwired: 1 in, 9 out]
          n109 = call <vilib>:"WPI_AnalogChannelGetVoltage.vi"("AIDeviceRef"=w56) -> ("Voltage"=w53:dbl)  [unwired: 1 in, 9 out]
          n110 = Subtract(x=w53, y=2.5) -> (x-y=w37:dbl)
          n111 = local read "ARM_REV_LIMIT"() -> (w33:dbl)
          n112 = Negate(x=w37) -> (-x=w38:dbl)
          n113 = Divide(x=w38, y=2.5) -> (x/y=w36:dbl)
          n114 = local read "ARM_FWD_LIMIT"() -> (w32:dbl)
          n115 = Greater?(x=w32, y=w36) -> (0:w49:bool)
          n116 = Less?(x=w33, y=w36) -> (x < y?=w50:bool)
          n117 = call-poly <vilib>:"PID.vi"("output range"=cluster{"output low":dbl, "output high":dbl} {"output low"=-0.75, "output high"=0.5}, "PID gains"=T3 {"proportional gain (Kc)"=3.0, "integral time (Ti, min)"=0.0, "derivative time (Td, min)"=0.0}, "process variable"=w36, "setpoint"=w34) -> ("output"=w42:dbl)  [unwired: 2 in, 5 out]
          n118 = Select(t=1.0, s=w49, f=0.0) -> (s? t:f=w47:dbl)
          n119 = Select(t=-1.0, s=w50, f=0.0) -> (s? t:f=w48:dbl)
          n120 = In Range and Coerce(upper limit=w47, x=w42, lower limit=w48) -> (coerced(x)=w35:dbl)  [unwired: 1 out]
          n121 = call <vilib>:"WPI_MotorControlRefNum Registry Get.vi"("refnum name"="Ball_Grabber_Arm") -> ("MotorControlDevRef"=w57:T5)  [unwired: 1 in, 9 out]
          n122 = Negate(x=w35) -> (-x=w39:dbl)
          n123 = local write "Feeder_Arm_Speed"(w39) -> ()
          n124 = call <vilib>:"WPI_MotorControlSetOutput.vi"("Output"=w39, "MotorControlDevRef"=w57) -> ()  [unwired: 3 in, 7 out]
        }
        frame Disabled {
        }
      }
    }
    frame Disabled {
    }
  }
  n125 = while {
    stop <- FALSE stop-if-true
    n126 = call <vilib>:"WPI_DriverStationReport Robot Code State.vi"("Autonomous"=TRUE) -> ()  [unwired: 10 in, 1 out]
    n127 = Wait (ms)(milliseconds to wait=u32 20) -> ()  [unwired: 1 out]
  }
  n128 = global write "Robot Global Data.vi" "LED toggle rate (ms)"(u32 500 ("LED ms toggle rate")) -> ()
  n129 = disable-structure shown="Disabled" {
    frame Disabled {
      # "This is some simple sample code to drive your robot.  When using the RobotDrive VIs, you must call them at least every 100ms.  Otherwise, for safety, your robot will be stopped and an error will be reported."
      # "stand still"
      # "turn left for 0.5 second"
      # "turn right for 1 second"
      n130 = call <vilib>:"WPI_RobotDriveRefNum Registry Get.vi"("refnum name"="Left and Right Motors") -> ("RobotDriveDevRef"=w618:T4)  [unwired: 1 in, 9 out]
      n131 = while {
        tunnel: w618 -> [w643]
        tunnel: [w636] -> w617
        i -> [w639]
        stop <- w637 stop-if-true
        n132 = Increment(x=w639) -> (x+1=w635:i32)
        n133 = Wait (ms)(milliseconds to wait=u32 50) -> ()  [unwired: 1 out]
        n134 = call-poly <vilib>:"WPI_RobotDriveArcadeDrive.vi"("Y axis value"=0.5 ("X axis value"), "X axis value"=0.25, "RobotDriveDevRef"=w643) -> ("RobotDriveDevRef"=w636:T4)  [unwired: 1 in, 7 out]
        n135 = Greater Or Equal?(x=w635, y=20) -> (x >= y?=w637:bool)
      }
      n136 = while {
        tunnel: w617 -> [w634]
        tunnel: [w627] -> w616
        i -> [w630]
        stop <- w628 stop-if-true
        n137 = Increment(x=w630) -> (x+1=w626:i32)
        n138 = Wait (ms)(milliseconds to wait=u32 50) -> ()  [unwired: 1 out]
        n139 = call-poly <vilib>:"WPI_RobotDriveArcadeDrive.vi"("Y axis value"=0.25 ("X axis value"), "X axis value"=0.5, "RobotDriveDevRef"=w634) -> ("RobotDriveDevRef"=w627:T4)  [unwired: 1 in, 7 out]
        n140 = Greater Or Equal?(x=w626, y=10) -> (x >= y?=w628:bool)
      }
      n141 = while {
        tunnel: w616 -> [w625]
        tunnel: [w621] -> _
        stop <- FALSE stop-if-true
        # "keep calling RobotDrive in a loop to avoid an error message"
        n142 = Wait (ms)(milliseconds to wait=u32 50) -> ()  [unwired: 1 out]
        n143 = call-poly <vilib>:"WPI_RobotDriveArcadeDrive.vi"("Y axis value"=0.0 ("X axis value"), "X axis value"=0.0, "RobotDriveDevRef"=w625) -> ("RobotDriveDevRef"=w621:T4)  [unwired: 1 in, 7 out]
      }
    }
    frame Enabled {
    }
  }
